vi "GetProtoParseError.vi"(8 "error in (no error)":errorcluster, 11 "Protofile ref in":u64) -> (0 "error out":errorcluster, 2 "Error Message":string, 3 "Protofile ref out":u64)   [LabVIEW 2019, in "gRPC Template Creation Utility.lvlib"]
uses:
  gRPC Template Creation Utility.lvlib
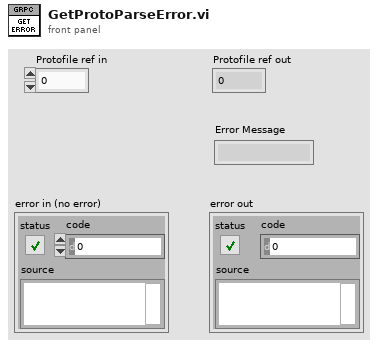
[diagram p1: front panel]
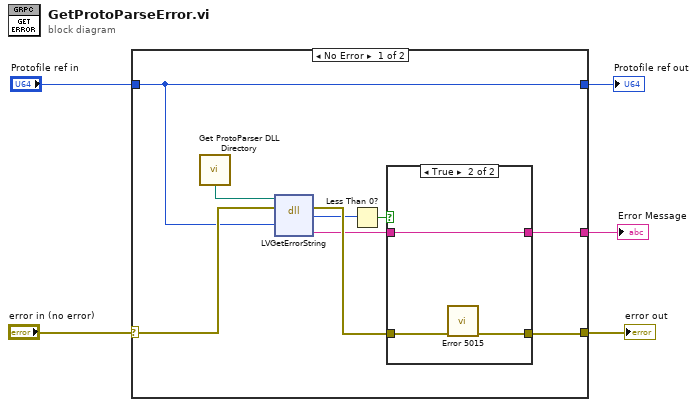
[diagram p0: block diagram]
diagram:
  n1 = case shown="No Error" "error in (no error)" {
    selector: "error in (no error)" -> [w13 w20]
    tunnel: "Protofile ref in" -> [w12 w21]
    tunnel: [w12 w21] -> w4
    tunnel: [w11 w20] -> w3
    tunnel: [w6 _] -> w1
    frame No Error {
      n2 = call "Get ProtoParser DLL Directory.vi"() -> ("Proto Parser Directory"=w14:path)
      n3 = dll-call lib="?" fn="LVGetErrorString"(path in=w14, error in=w13, "protoDescription"=w12) -> (error out=w10:errorcluster, "return type"=w9:i32, "ErrorMessage"=w7:string)  [unwired: 3 in, 1 out]
      n4 = Less Than 0?(x=w9) -> (x < 0?=w8:bool)
      n5 = case shown="True" w8 {
        tunnel: [w15 w19] -> w11
        tunnel: w10 -> [w15 w18]
        tunnel: w7 -> [w16 w17]
        tunnel: [w16 w17] -> w6
        frame False {
        }
        frame True {
          n6 = call "Error 5015.vi"("error in (no error)"=w18) -> ("error out"=w19:errorcluster)  [unwired: 10 in]
        }
      }
    }
    frame Error {
    }
  }
  "Protofile ref out" <- w4
  "error out" <- w3
  "Error Message" <- w1
